vi "Number.vi"(8 "Error In":errorcluster, 10 "Number":dbl, 11 "CS++RTMainActor in":refnum<class "CS++RTMainActor.lvclass">) -> (0 "Error Out":errorcluster, 3 "CS++RTMainActor out":refnum<class "CS++RTMainActor.lvclass">)   [LabVIEW 2016]
doc: "Set attribute attribute and publish to SV."
uses:
  CS++RTMainActor.lvclass
  C:/Program Files (x86)/National Instruments/LabVIEW 2016/vi.lib/ActorFramework/Actor/Actor.lvclass
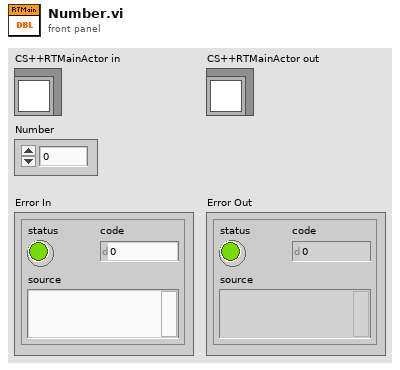
[diagram p1: front panel]
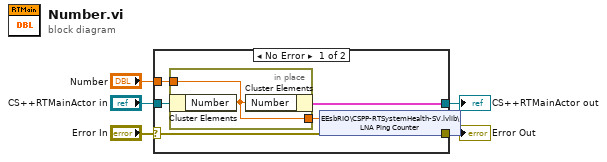
[diagram p0: block diagram]
diagram:
  n1 = case shown="No Error" "Error In" {
    selector: "Error In" -> [w8 w14]
    tunnel: [w7 w14] -> w2
    tunnel: [w10 w13] -> w4
    tunnel: "CS++RTMainActor in" -> [w11 w13]
    tunnel: "Number" -> [w6 _]
    frame No Error {
      n2 = in-place {
        in-place-border: [w12] -> w9
        in-place-border: w6 -> [w12]
        n3 = in-place-cluster #1(w11) -> ()  [unwired: 1 out]
        n4 = in-place-cluster #1("Number"=w12) -> (w10:cluster{})
      }
      n5 = shared-variable "EEsbRIO\\CSPP-RTSystemHealth-SV.lvlib\\LNA Ping Counter"(w9, error in=w8) -> (error out=w7:errorcluster)
    }
    frame Error {
    }
  }
  "Error Out" <- w2
  "CS++RTMainActor out" <- w4
